vi "crane_under_load_monitor.vi"() -> ()   [LabVIEW 2024]
panel:
  out "l5_ground_pressure":sgl(slide) scale format="%.3f"
  out "l4_ground_pressure":sgl(slide) scale format="%.3f"
  out "l3_ground_pressure":sgl(slide) scale format="%.3f"
  out "l2_ground_pressure":sgl(slide) scale format="%.3f"
  out "l1_ground_pressure":sgl(slide) scale format="%.3f"
  out "error out":errorcluster
  in  "stop":bool
  out "period(Hz)":dbl(knob) scale=0.0..40.0
  out "l5_gp_max":bool
  out "l4_gp_max":bool
  out "l3_gp_max":bool
  out "l2_gp_max":bool
  out "l1_gp_max":bool
  out "r5_gp_max":bool
  out "r4_gp_max":bool
  out "r3_gp_max":bool
  out "r2_gp_max":bool
  out "r1_gp_max":bool
  out "MaxGroundPressure":T1(graph)
  out "Load_state":sgl(graph)
  out "Angle":T2(graph)
  in  "Load(ton)":sgl(slide)=40.0 scale=40.0..120.0
  in  "boom_angle(degree)":sgl(knob)=40.0 scale=40.0..70.0 scale format="%_1f"
  in  "swing_angle(degree)":sgl(knob) scale=0.0..180.0 scale format="%_1f"
  out "r5_ground_pressure":sgl(slide) scale=0.0..500.0 scale format="%.3f"
  out "r4_ground_pressure":sgl(slide) scale=0.0..500.0 scale format="%.3f"
  out "r3_ground_pressure":sgl(slide) scale=0.0..500.0 scale format="%.3f"
  out "r2_ground_pressure":sgl(slide) scale=0.0..500.0 scale format="%.3f"
  out "r1_ground_pressure":sgl(slide) scale=0.0..500.0 scale format="%.3f"
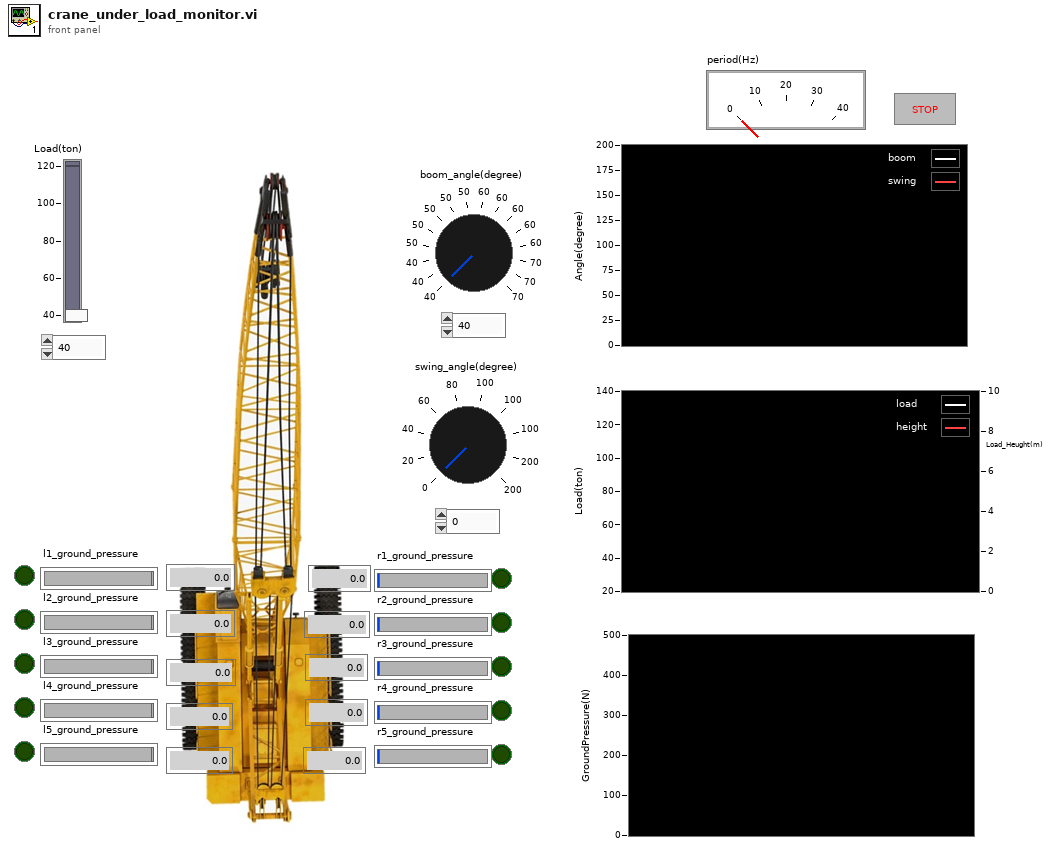
[diagram p1: front panel]
types:
  T1 = cluster{sgl, sgl, sgl, sgl, sgl, sgl, sgl, sgl, sgl, sgl}
  T2 = cluster{"boom_angle(degree)":sgl, "swing_angle(degree)":sgl}
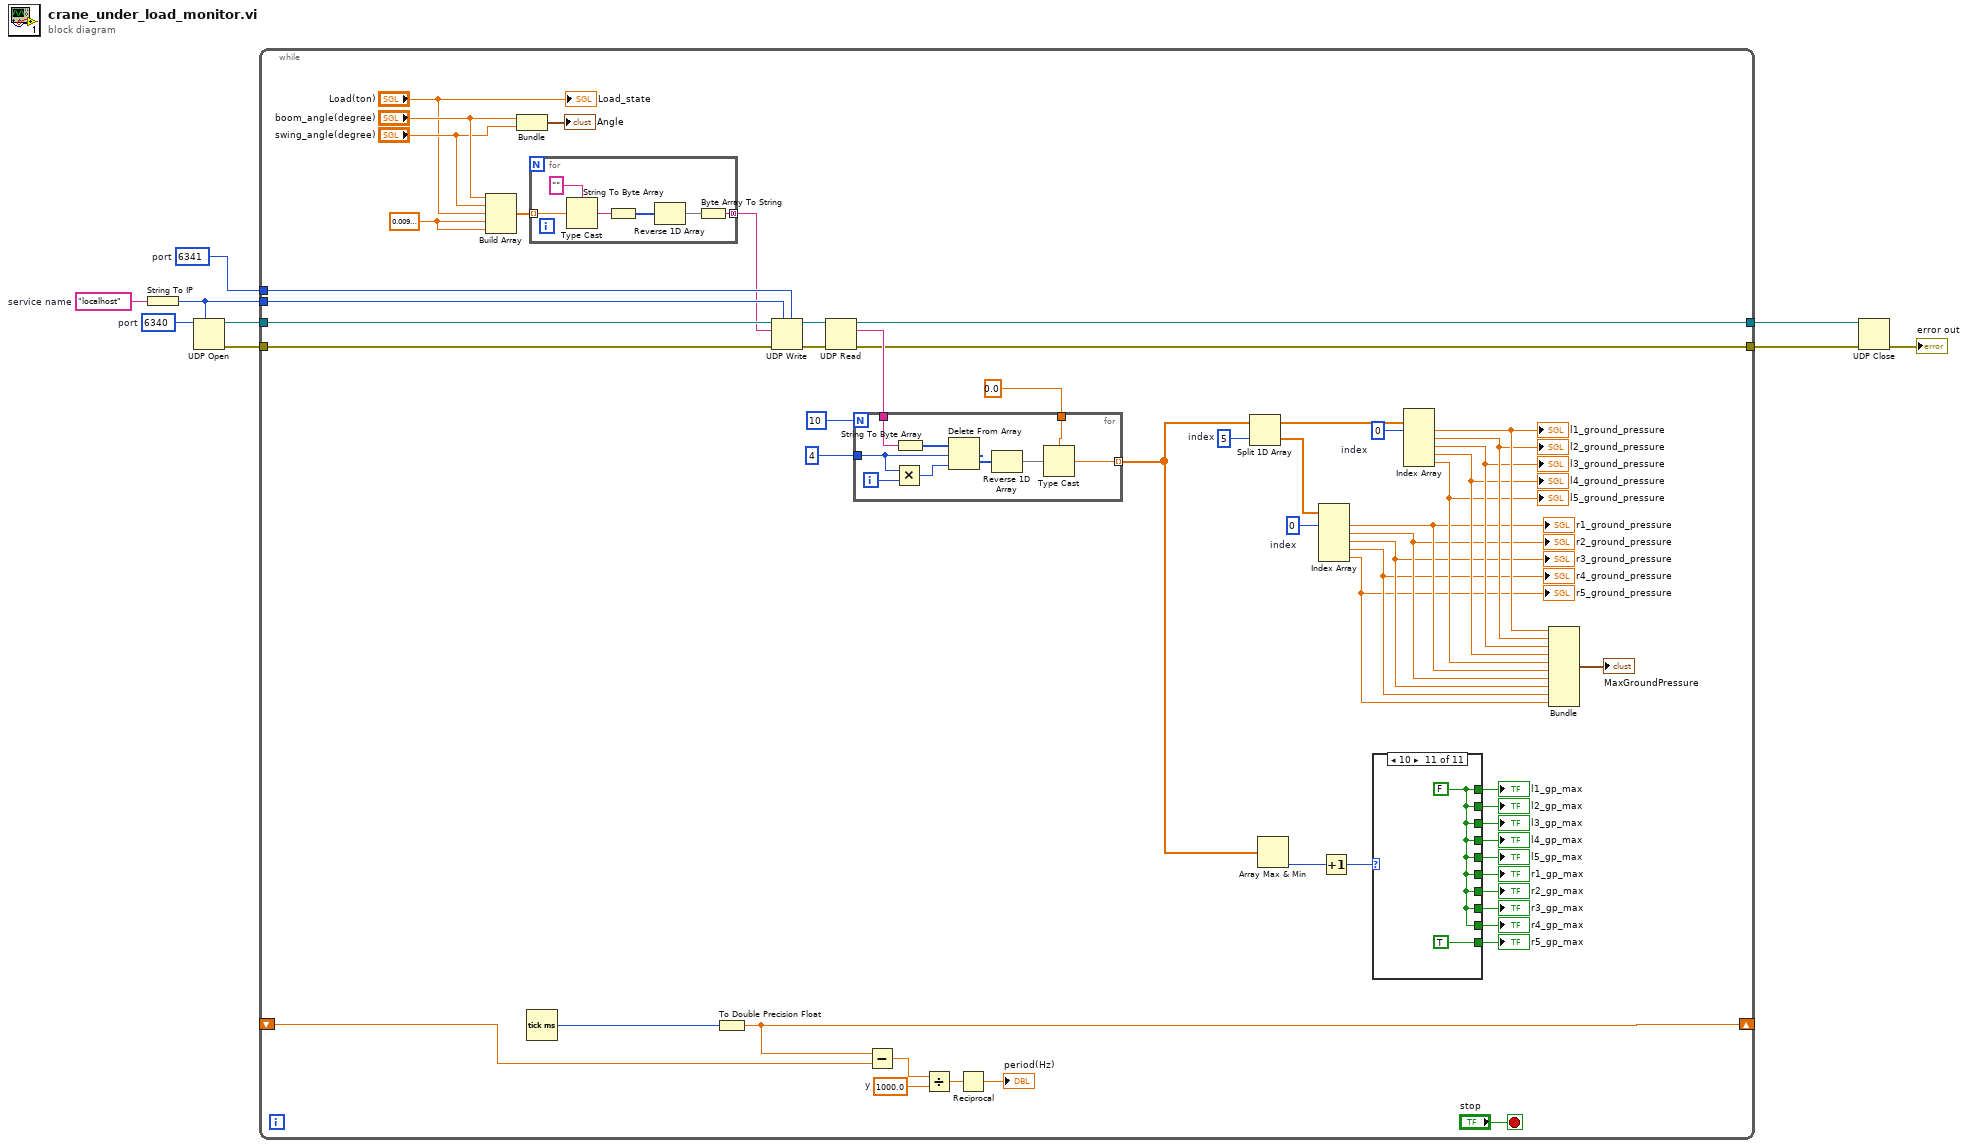
[diagram p0: block diagram]
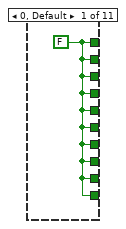
[diagram p2: hidden frame]
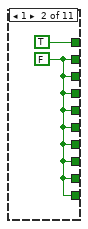
[diagram p3: hidden frame]
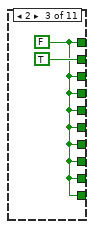
[diagram p4: hidden frame]
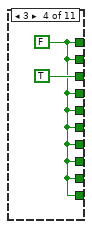
[diagram p5: hidden frame]
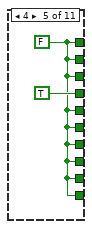
[diagram p6: hidden frame]
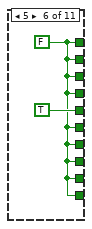
[diagram p7: hidden frame]
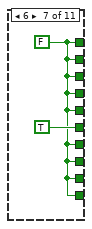
[diagram p8: hidden frame]
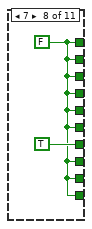
[diagram p9: hidden frame]
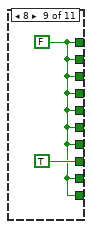
[diagram p10: hidden frame]
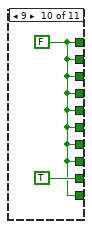
[diagram p11: hidden frame]
diagram:
  w3 = u16 6341  # port
  w7 = "localhost"  # service name
  w6 = u16 6340  # port
  n1 = String To IP(1:w7) -> (0:w2:u32)
  n2 = UDP Open(7:w2, 11:w6) -> (port=w5:refnum<k16>, 0:w4:errorcluster)  [unwired: 3 in, 1 out]
  n3 = while {
    tunnel: [w29] -> w9
    shift-right: [w49] -> _
    shift-left: _ -> [w48]
    tunnel: w5 -> [w21]
    tunnel: w4 -> [w20]
    tunnel: w2 -> [w18]
    tunnel: w3 -> [w19]
    tunnel: [w11] -> w1
    stop <- "stop" stop-if-true
    w10 = sgl 0.01 ("element")
    w43 = 0  # index
    w45 = 5  # index
    w52 = 1000.0  # y
    w54 = 0  # index
    n4 = Build Array("boom_angle(degree)", "swing_angle(degree)", "Load(ton)", w10, w10) -> (w24:sgl[])
    n5 = Bundle("boom_angle(degree)"="boom_angle(degree)", "swing_angle(degree)"="swing_angle(degree)") -> (→"Angle":T2)  [unwired: 1 in]
    n6 = Tick Count (ms)() -> (millisecond timer value=w50:u32)
    n7 = for {
      tunnel: w24 -> [w80] mode=indexing
      tunnel: [w75] -> w17 mode=concatenating
      n8 = Type Cast(type="" ("data out"), x=w80) -> (*(type *) &x=w78:string)
      n9 = String To Byte Array(string=w78) -> (unsigned byte array=w77:u8[])
      n10 = Reverse 1D Array(array=w77) -> (reversed array=w76:u8[])
      n11 = Byte Array To String(unsigned byte array=w76) -> (string=w75:string)
    }
    n12 = To Double Precision Float(number=w50) -> (double precision float=w49:dbl)
    n13 = UDP Write(address=w18, port or service name=w19, connection ID=w21, data in=w17, 8:w20) -> (error out=w22:errorcluster, 3:w23:refnum<k16>)  [unwired: 1 in]
    n14 = UDP Read(connection ID=w23, 8:w22) -> (data out=w16:string, error out=w11:errorcluster, 3:w29:refnum<k16>)  [unwired: 2 in, 2 out]
    n15 = for {
      N: 10 -> [_]
      tunnel: w16 -> [w74]
      tunnel: 4 ("length") -> [w71]
      tunnel: sgl 0.0 -> [w67]
      tunnel: [w66] -> w12 mode=indexing
      i -> [w72]
      n16 = Multiply(x=w71, y=w72) -> (x*y=w70:i32)
      n17 = String To Byte Array(string=w74) -> (unsigned byte array=w73:u8[])
      n18 = Delete From Array(array=w73, length=w71, index=w70) -> (deleted portion=w69:u8[])  [unwired: 1 out]
      n19 = Reverse 1D Array(array=w69) -> (reversed array=w68:u8[])
      n20 = Type Cast(type=w67, x=w68) -> (*(type *) &x=w66:sgl)
    }
    n21 = Subtract(x=w49, y=w48) -> (x-y=w53:dbl)
    n22 = Divide(x=w53, y=w52) -> (x/y=w51:dbl)
    n23 = Reciprocal(x=w51) -> (1/x=→"period(Hz)":dbl)
    n24 = Split 1D Array(array=w12, index=w45) -> (first subarray=w42:sgl[], second subarray=w44:sgl[])
    n25 = Array Max & Min(array=w12) -> (min index (indices)=w30:i32)  [unwired: 3 out]
    n26 = Index Array(array=w44, index #1=w43) -> (element #1=w36:sgl, element #2=w35:sgl, element #3=w34:sgl, element #4=w33:sgl, element #5=w32:sgl)  [unwired: 4 in]
    "r1_ground_pressure" <- w36
    "r2_ground_pressure" <- w35
    "r3_ground_pressure" <- w34
    "r4_ground_pressure" <- w33
    "r5_ground_pressure" <- w32
    n27 = Increment(x=w30) -> (x+1=w55:i32)
    n28 = case shown="10" w55 {
      tunnel: [w81 TRUE w84 w86 w88 w90 w92 w94 w96 w98 w100] -> w65
      tunnel: [w81 w82 TRUE w86 w88 w90 w92 w94 w96 w98 w100] -> w64
      tunnel: [w81 w82 w84 TRUE w88 w90 w92 w94 w96 w98 w100] -> w63
      tunnel: [w81 w82 w84 w86 TRUE w90 w92 w94 w96 w98 w100] -> w62
      tunnel: [w81 w82 w84 w86 w88 TRUE w92 w94 w96 w98 w100] -> w61
      tunnel: [w81 w82 w84 w86 w88 w90 TRUE w94 w96 w98 w100] -> w60
      tunnel: [w81 w82 w84 w86 w88 w90 w92 TRUE w96 w98 w100] -> w59
      tunnel: [w81 w82 w84 w86 w88 w90 w92 w94 TRUE w98 w100] -> w58
      tunnel: [w81 w82 w84 w86 w88 w90 w92 w94 w96 TRUE w100] -> w57
      tunnel: [w81 w82 w84 w86 w88 w90 w92 w94 w96 w98 TRUE] -> w56
      frame 0, Default {
        w81 = FALSE
      }
      frame 1 {
        w82 = FALSE
      }
      frame 2 {
        w84 = FALSE
      }
      frame 3 {
        w86 = FALSE
      }
      frame 4 {
        w88 = FALSE
      }
      frame 5 {
        w90 = FALSE
      }
      frame 6 {
        w92 = FALSE
      }
      frame 7 {
        w94 = FALSE
      }
      frame 8 {
        w96 = FALSE
      }
      frame 9 {
        w98 = FALSE
      }
      frame 10 {
        w100 = FALSE
      }
    }
    "r1_gp_max" <- w60
    "r2_gp_max" <- w59
    "r3_gp_max" <- w58
    "r4_gp_max" <- w57
    "r5_gp_max" <- w56
    "l1_gp_max" <- w65
    "l2_gp_max" <- w64
    "l3_gp_max" <- w63
    "l4_gp_max" <- w62
    "l5_gp_max" <- w61
    n29 = Index Array(array=w42, index #1=w54) -> (element #1=w41:sgl, element #2=w40:sgl, element #3=w39:sgl, element #4=w38:sgl, element #5=w37:sgl)  [unwired: 4 in]
    "l1_ground_pressure" <- w41
    "l2_ground_pressure" <- w40
    "l3_ground_pressure" <- w39
    "l4_ground_pressure" <- w38
    "l5_ground_pressure" <- w37
    n30 = Bundle(w41, w40, w39, w38, w37, w36, w35, w34, w33, w32) -> (→"MaxGroundPressure":T1)  [unwired: 1 in]
    "Load_state" <- "Load(ton)"
  }
  n31 = UDP Close(connection ID=w9, 8:w1) -> (error out=→"error out":errorcluster)  [unwired: 1 out]
